vi "Check for Valid Steering Frame.vi"(7 "produce error if invalid (T)":bool=TRUE, 8 "error in (no error)":errorcluster, 11 "steering frame in":refnum<class "NI_Robotics_Steering Frame.lvclass">) -> (0 "error out":errorcluster, 2 "valid?":bool, 3 "steering frame out":refnum<class "NI_Robotics_Steering Frame.lvclass">)   [LabVIEW 2017, in "NI_Robotics_Steering Frame.lvclass"]
uses:
  <vilib>/robotics/Steering/Steering Frame/NI_Robotics_Steering Frame.lvclass
  <vilib>/robotics/Steering/Steering Frame/NI_Robotics_Steering Frame.lvclass/NI_Robotics_Steering Frame.ctl
  <vilib>/robotics/Utilities/NI_Robotics Utilities.lvlib
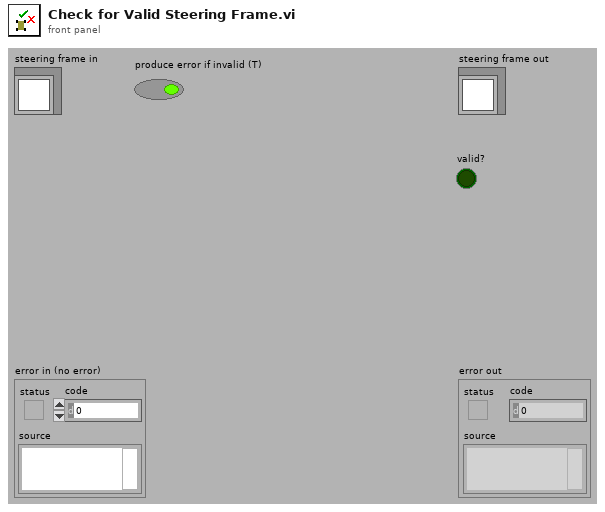
[diagram p1: front panel]
types:
  T1 = typedef "NI_Robotics_Steering Frame.lvclass/Wheel Orientation.ctl" = cluster{"wheel":refnum<class "NI_Robotics_Wheel.lvclass">, "x position":dbl, "y position":dbl, "frame angle (rad)":dbl}
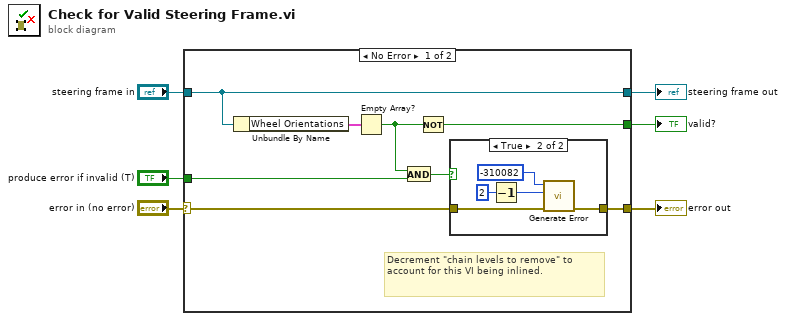
[diagram p0: block diagram]
diagram:
  n1 = case shown="No Error" "error in (no error)" {
    selector: "error in (no error)" -> [w8 w22]
    tunnel: [w7 w22] -> w5
    tunnel: [w14 w21] -> w3
    tunnel: "steering frame in" -> [w14 w21]
    tunnel: "produce error if invalid (T)" -> [w12 _]
    tunnel: [w10 _] -> w1
    frame No Error {
      # "Decrement \"chain levels to remove\" to account for this VI being inlined."
      n2 = Unbundle By Name(w14) -> ("Wheel Orientations"=w13:T1[])
      n3 = Empty Array?(array=w13) -> (empty?=w11:bool)
      n4 = And(x=w11, y=w12) -> (x .and. y?=w9:bool)
      n5 = Not(x=w11) -> (.not. x?=w10:bool)
      n6 = case shown="True" w9 {
        tunnel: w8 -> [w15 w20]
        tunnel: [w15 w19] -> w7
        frame False {
        }
        frame True {
          n7 = Decrement(x=2 ("chain levels to remove (1)")) -> (x-1=w16:i32)
          n8 = call <vilib>:"Generate Error.vi"("error in (no error)"=w20, "chain levels to remove (1)"=w16, "code"=-310082) -> ("error out"=w19:errorcluster)  [unwired: 8 in]
        }
      }
    }
    frame Error {
    }
  }
  "error out" <- w5
  "steering frame out" <- w3
  "valid?" <- w1
